vi "Byte_data_변환.vi"() -> ()   [LabVIEW 2017]
panel:
  out "불리언":bool
  out "배열":i32[](array[numeric])
  out "숫자형 컨트롤 2":i32
  out "unsigned byte array":u8[][](array[numeric])
  out "숫자형 컨트롤":i32
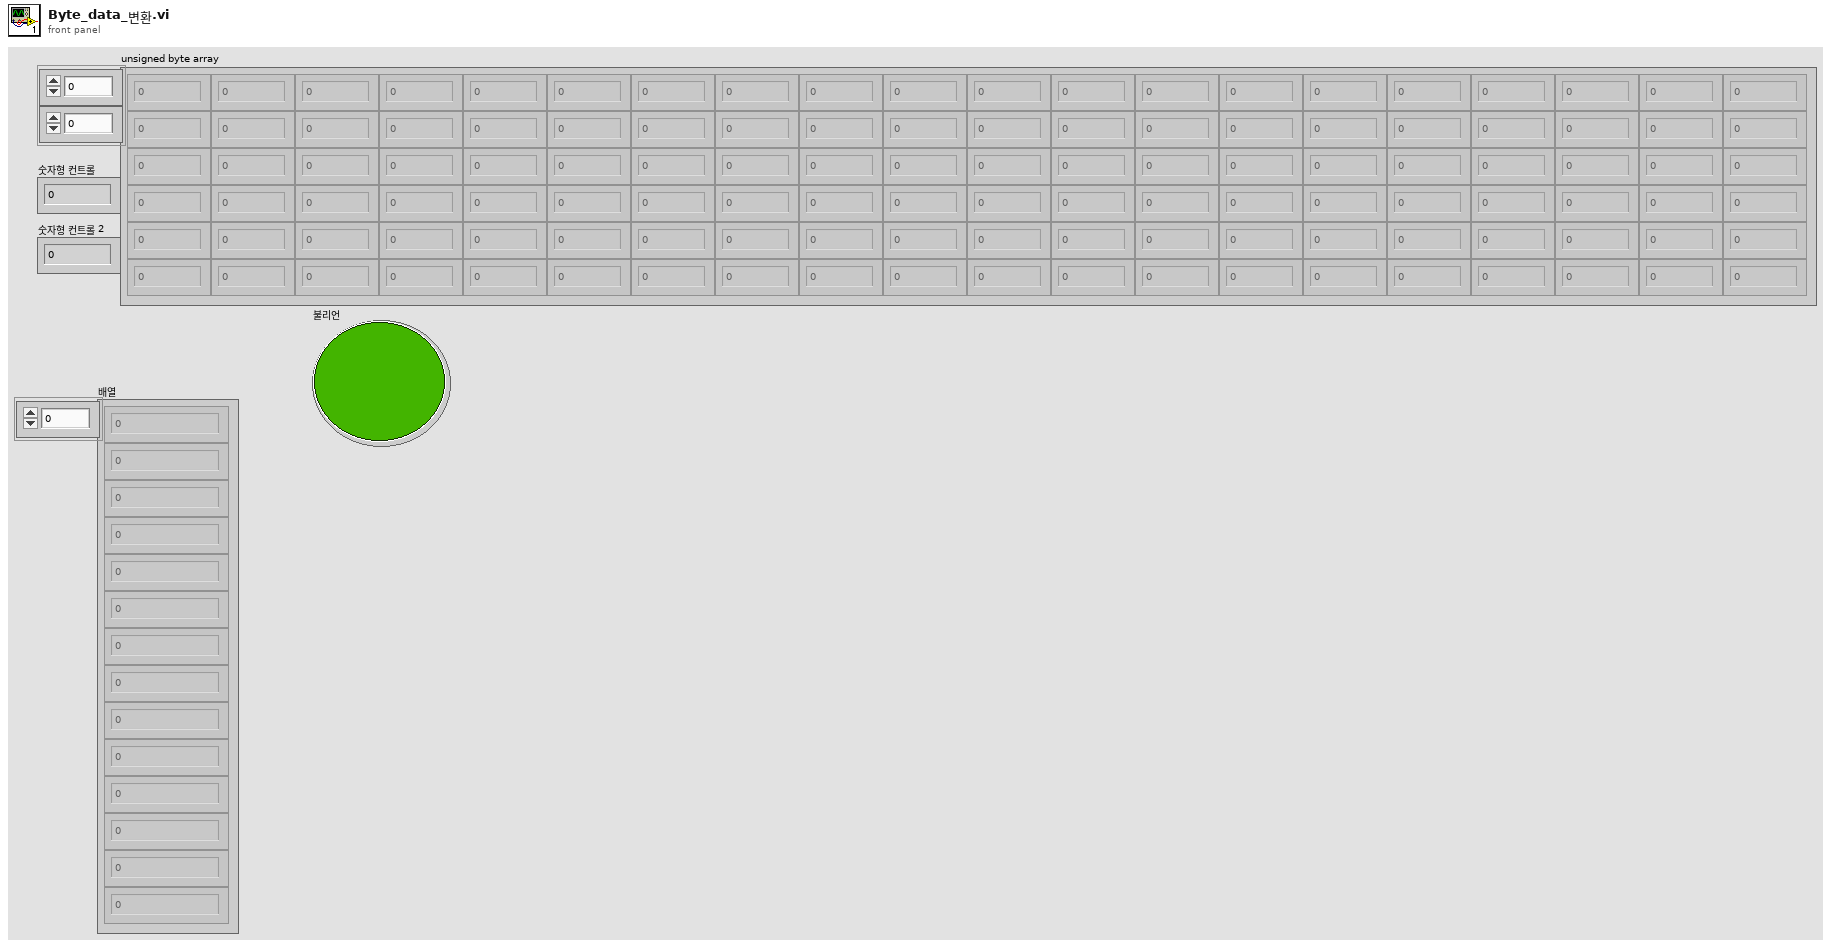
[diagram p1: front panel]
types:
  T1 = enum16{"Standard", "Buffered", "CRLF", "Immediate"}
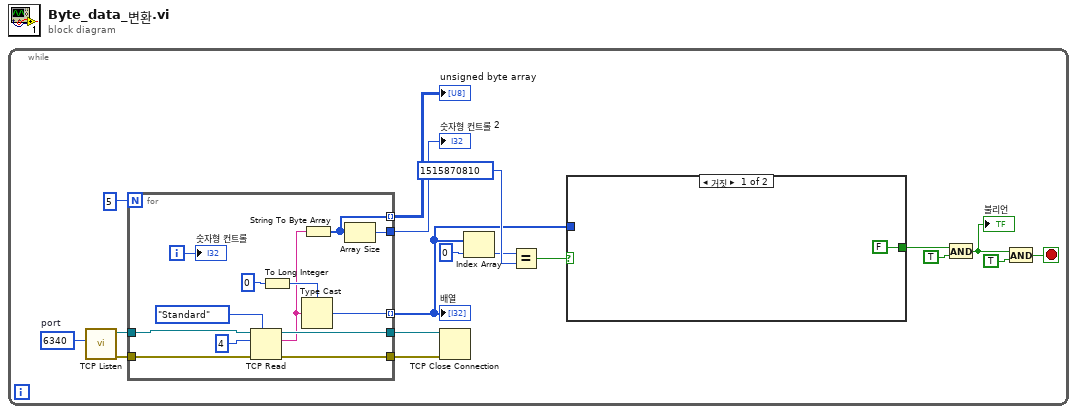
[diagram p0: block diagram]
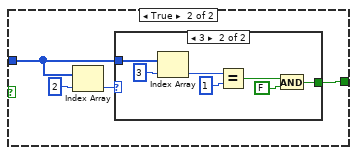
[diagram p2: hidden frame]
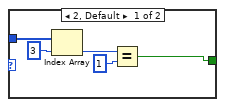
[diagram p3: hidden frame]
diagram:
  n1 = while {
    stop <- w1 stop-if-true
    w14 = u16 6340  # port
    n2 = call <vilib>:"TCP Listen.vi"("port"=w14) -> ("error out"=w17:errorcluster, "connection ID"=w18:refnum<k5>)  [unwired: 6 in, 3 out]
    n3 = for {
      N: 5 -> [_]
      tunnel: w18 -> [w48]
      tunnel: w17 -> [w47]
      tunnel: [w46] -> w16
      tunnel: [w40] -> w15
      tunnel: [w42] -> w12 mode=indexing
      tunnel: [w41] -> w11
      tunnel: [w36] -> w6 mode=indexing
      i -> [w43]
      n4 = TCP Read(connection ID=w48, bytes to read=4 ("읽을 바이트"), error in (no error)=w47, 7:T1."Standard" ("모드(standard)")) -> (connection ID out=w46:refnum<k5>, data out=w37:string, error out=w40:errorcluster)  [unwired: 1 out]
      n5 = To Long Integer(number=0 ("숫자")) -> (32bit integer=w39:i32)
      n6 = Type Cast(type=w39, x=w37) -> (*(type *) &x=w36:i32)
      n7 = String To Byte Array(string=w37) -> (unsigned byte array=w42:u8[])
      n8 = Array Size(array=w42) -> (size(s)=w41:i32)
      "숫자형 컨트롤" <- w43
    }
    "unsigned byte array" <- w12
    "숫자형 컨트롤 2" <- w11
    "배열" <- w6
    n9 = TCP Close Connection(connection ID=w16, error in (no error)=w15) -> ()  [unwired: 3 out]
    n10 = Index Array(array=w6, index=0 ("인덱스")) -> (element=w8:i32)
    n11 = Equal?(x=w8, y=1515870810) -> (x = y?=w7:bool)
    n12 = case shown="거짓" w7 {
      tunnel: w6 -> [_ w21]
      tunnel: [FALSE w20] -> w5
      frame False {
      }
      frame True {
        n13 = Index Array(array=w21, index=2 ("인덱스")) -> (element=w22:i32)
        n14 = case shown="3" w22 {
          tunnel: w21 -> [w28 w35]
          tunnel: [w24 w29] -> w20
          frame 2, Default {
            n15 = Index Array(array=w28, index=3 ("인덱스")) -> (element=w26:i32)
            n16 = Equal?(x=w26, y=1) -> (x = y?=w24:bool)
          }
          frame 3 {
            n17 = Index Array(array=w35, index=3 ("인덱스")) -> (element=w33:i32)
            n18 = Equal?(x=w33, y=1) -> (x = y?=w31:bool)
            n19 = And(x=w31, y=FALSE) -> (x .and. y?=w29:bool)
          }
        }
      }
    }
    n20 = And(x=w5, y=TRUE) -> (x .and. y?=w3:bool)
    "불리언" <- w3
    n21 = And(x=w3, y=TRUE) -> (x .and. y?=w1:bool)
  }
